vi "clearplot.vi"(8 "error in (no error)":errorcluster, 10 "plotnum":i32, 11 "Automation Refnum in":refnum<k7>) -> (0 "error out":errorcluster, 3 "Automation Refnum out":refnum<k7>)   [LabVIEW 2015]
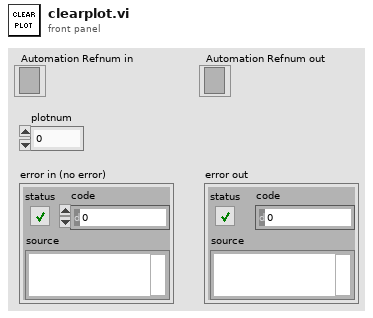
[diagram p1: front panel]
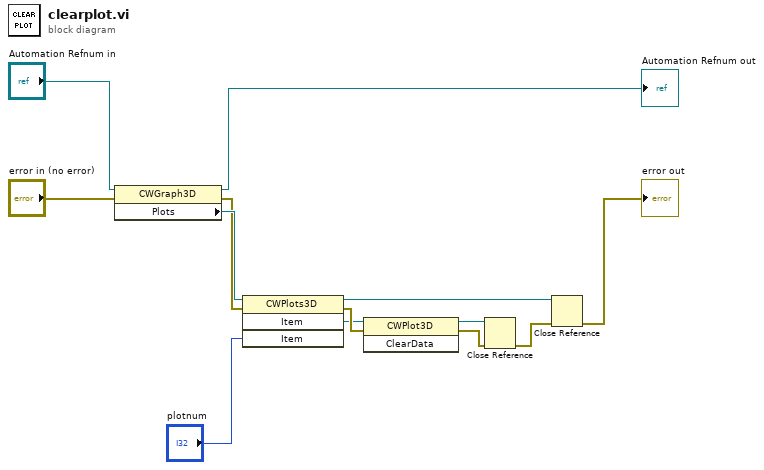
[diagram p0: block diagram]
diagram:
  n1 = property class="CWGraph3D"(reference="Automation Refnum in", error in="error in (no error)") -> (reference out=→"Automation Refnum out":refnum<k7>, error out=w3:errorcluster, "Plots"=w4:refnum<k7>)
  n2 = invoke class="CWPlots3D" method="Item"(reference=w4, error in=w3, "Item"="plotnum") -> (reference out=w11:refnum<k7>, error out=w7:errorcluster, "Item"=w6:refnum<k7>)  [unwired: 1 in, 1 out]
  n3 = invoke class="CWPlot3D" method="ClearData"(reference=w6, error in=w7) -> (reference out=w9:refnum<k7>, error out=w8:errorcluster)  [unwired: 1 in, 1 out]
  n4 = Close Reference(reference=w9, error in (no error)=w8) -> (error out=w10:errorcluster)
  n5 = Close Reference(reference=w11, error in (no error)=w10) -> (error out=→"error out":errorcluster)
